vi "TharShutDown.vi"(8 "error in (no error)":errorcluster, 11 "Device Serial Number":string) -> (0 "Error Out":errorcluster, 3 "Device Serial Number Out":string)   [LabVIEW 2016]
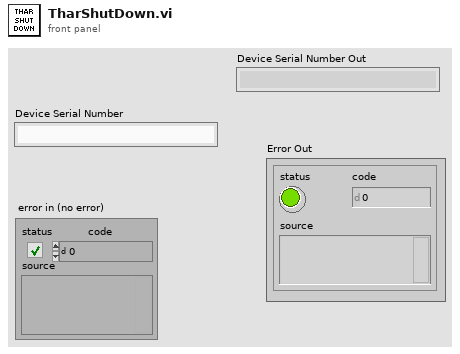
[diagram p1: front panel]
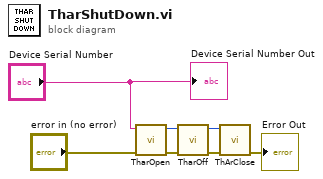
[diagram p0: block diagram]
diagram:
  n1 = call "TharOpen.vi"("error in (no error)"="error in (no error)", "Device Serial Number"="Device Serial Number") -> ("error constant"=w6:errorcluster, "Handle"=w7:u32)  [unwired: 8 in]
  n2 = call "TharOff.vi"("Error In"=w6, "Handle In"=w7) -> ("Error Out"=w2:errorcluster, "Handle Out"=w3:u32)  [unwired: 8 in]
  n3 = call "ThArClose.vi"("error in (no error)"=w2, "Handle"=w3) -> ("error out"=→"Error Out":errorcluster)  [unwired: 9 in]
  "Device Serial Number Out" <- "Device Serial Number"
